vi "Debug.vi"() -> ()   [LabVIEW 2018, in "Globals.lvlib"]
uses:
  Globals.lvlib
panel:
  in  "Audio Transfer Latency (ms)":dbl
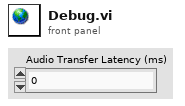
[diagram p1: front panel]
diagram:
